vi "CalcSingleSample.vi"(8 "error in (no error)":errorcluster, 11 "MultiBandState in":refnum<class "MultiBandState.lvclass">) -> (0 "error out":errorcluster, 3 "MultiBandState out":refnum<class "MultiBandState.lvclass">)   [LabVIEW 2014, in "Functions.lvlib" / "MultiBandState.lvclass"]
uses:
  MultiBandState.lvclass
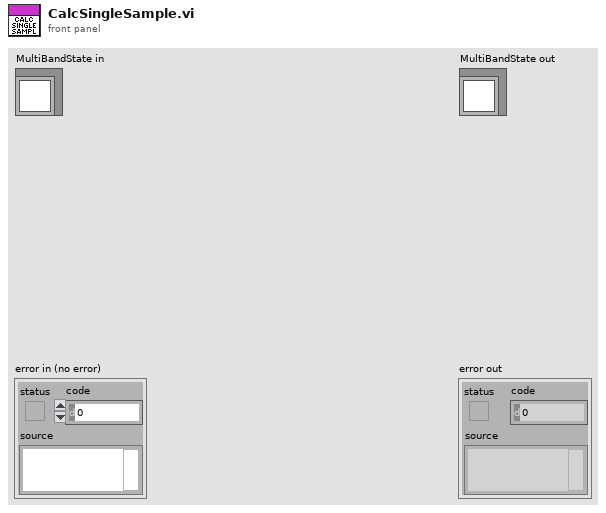
[diagram p1: front panel]
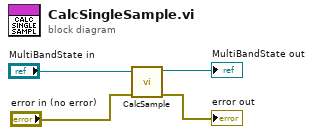
[diagram p0: block diagram]
diagram:
  n1 = call "CalcSample.vi"("error in (no error)"="error in (no error)", "MultiBandState in"="MultiBandState in") -> ("error out"=→"error out":errorcluster, "MultiBandState out"=→"MultiBandState out":refnum<class "MultiBandState.lvclass">)  [unwired: 8 in]
